vi "总氮质控流程.vi"(6 "队列输入TN":refnum<queue>, 9 "总氮":bool, 10 "总氮量程切换":enum32{"H", "L", "AUTO"}(ring)=enum."AUTO") -> (2 "总氮中断报警":bool, 3 "布尔":bool)   [LabVIEW 2016]
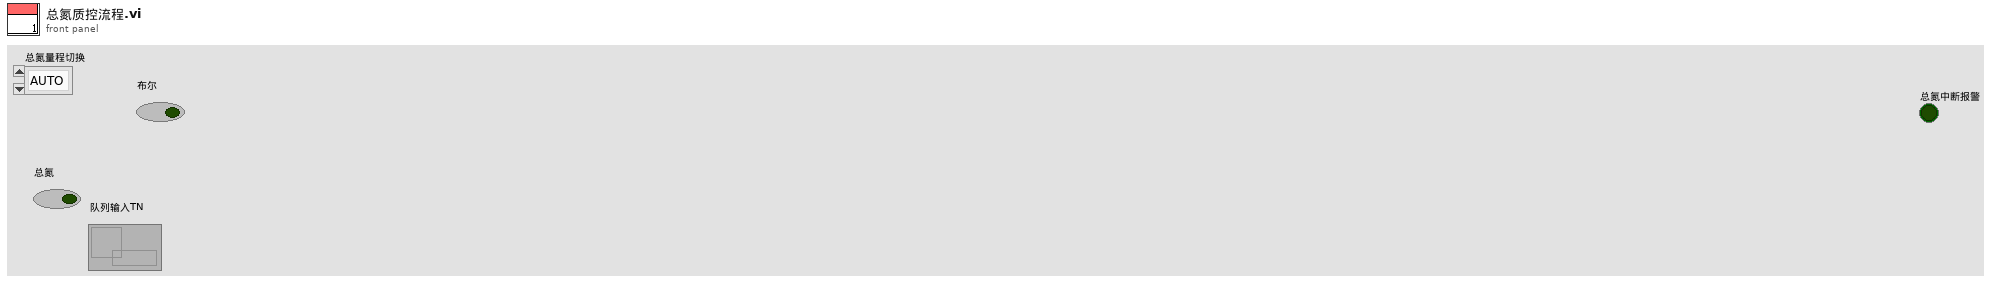
[diagram p1: front panel]
types:
  T1 = enum16{"待机", "启动氨氮水样", "氨氮测量中", "启动氨氮加标", "启动氨氮加标回收", "氨氮加标回收测量中", "启动总氮水样", "总氮测量中", "启动总氮加标", "启动总氮加标回收", "总氮加标回收测量中", "启动总磷水样", "总磷水样测量中", "启动总磷加标", "启动总磷加标回收", "总磷加标回收测量中", "结束"}
  T2 = cluster{"站号":u16, "量程切换":enum32{"H", "L", "AUTO"}, "控制命令":enum16{"启动测量", "标样核查", "零点核查", "跨度核查", "空白测试", "平行样测试", "加标回收", "空白校准", "标样校准", "初始化（清洗）", "停止测试", "仪器重启", "校时", "模式设置", "测量间隔设置"}, "模式设置":enum16{"待机", "连续模式", "周期模式", "定点模式", "受控模式", "手动模式"}, "测量间隔":u16}
  T3 = cluster{"时间标识":timestamp, "设备":string, "日志信息":string}
  T4 = cluster{"系统时间":timestamp, "工作状态":enum16{"空闲", "水样测试", "标样核查", "零点核查", "跨度核查", "空白测试", "平行样测试", "加标回收", "空白校准", "标样校准", "初始化（清洗）"}, "测量模式":enum16{"待机", "连续模式", "周期模式", "定点模式", "受控模式", "手动模式"}, "告警代码":enum16{"无告警", "缺试剂告警", "缺水样告警", "缺蒸馏水告警", "缺标液告警", "仪表漏液告警", "标定异常告警", "超量程告警", "加热异常", "低试剂预警", "超上限告警", "超下限告警", "仪表内部其他异常", "滴定异常告警", "电极异常告警", "量程切换告警", "参数设置告警", "PH电极电位异常", "电导率电极异常", "浊度光度异常", "溶解氧电极异常", "溶解氧光强异常", "温度异常告警", "PH异常告警", "溶解氧异常告警", "电导率异常告警", "浊度异常告警", "叶绿素异常告警", "藻密度异常告警", "蓝绿藻异常告警", "ORP异常告警", "氨氮异常告警", "清洁刷异常告警", "SD卡异常告警", "蓝牙异常告警", "Wifi异常告警", "流程异常告警"}, "故障代码":enum16{"无故障", "电机故障", "温度故障", "通讯故障", "滴定故障"}, "日志代码":u16, "软件版本":u16, "F0":sgl, "F1":sgl, "F2":sgl, "F3":sgl, "T":sgl, "H":sgl, "id":u16, "flowid":u16, "量程":u16, "总磷控温温度1":sgl, "营养盐控温温度2":sgl, "ADC":sgl}
  T5 = enum16{"空闲", "水样测试", "标样核查", "零点核查", "跨度核查", "空白测试", "平行样测试", "加标回收", "空白校准", "标样校准", "初始化（清洗）"}
  T6 = cluster{"因子编码":u32, "单位":u16, "标样参考值":sgl, "水样数据时间":timestamp, "水样实测值":sgl, "水样数据标识":string, "标样数据时间":timestamp, "标样实测值":sgl, "标样数据标识":string, "空白数据时间":timestamp, "空白实测值":sgl, "空白数据标识":string, "零点核查数据时间":timestamp, "零点核查实测值":sgl, "零点核查数据标识":string, "跨度核查数据时间":timestamp, "跨度核查实测值":sgl, "跨度核查数据标识":string, "加标回收数据时间":timestamp, "加标回收实测值":sgl, "加标回收数据标识":string, "平行样数据时间":timestamp, "平行样实测值":sgl, "平行样数据标识":string}
  T7 = cluster{"量程":dbl, "检出限":dbl, "加标前水样浓度":dbl, "加标后水样浓度":dbl, "加标水杯定容体积":dbl, "加标母液浓度":dbl, "加标体积":dbl, "加标回收率":dbl}
  T8 = cluster{"氨氮":u8, "总磷":u8, "总氮":u8, "CODMn":u8, "CODCr":u8}
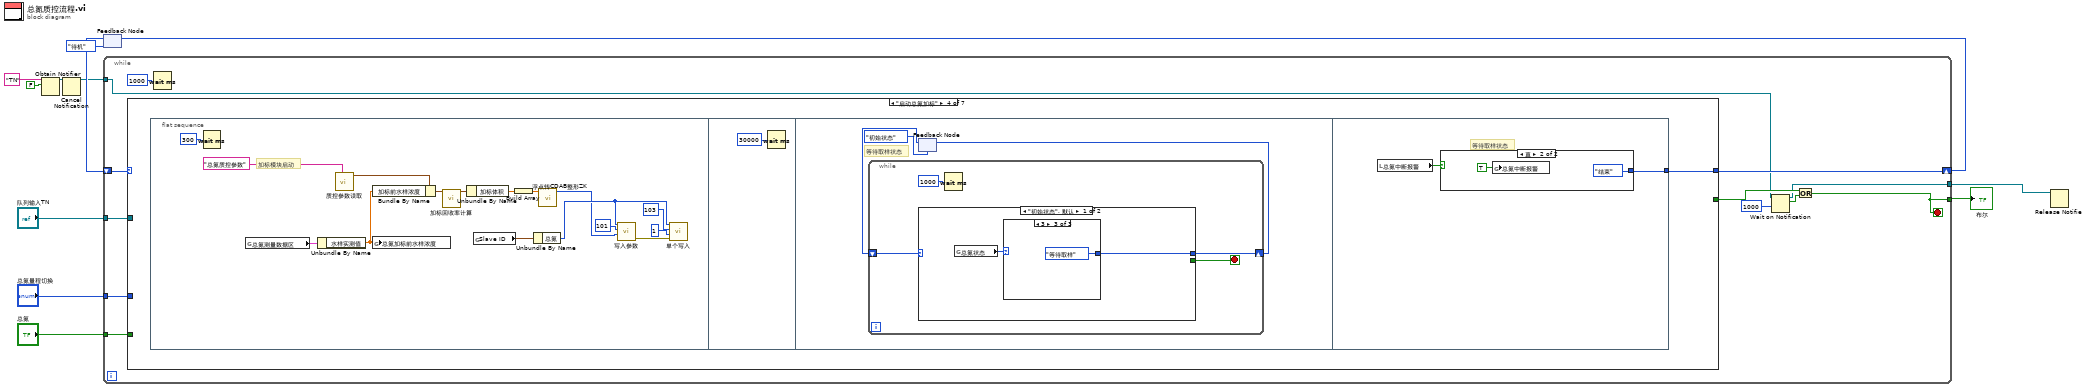
[diagram p0: block diagram]
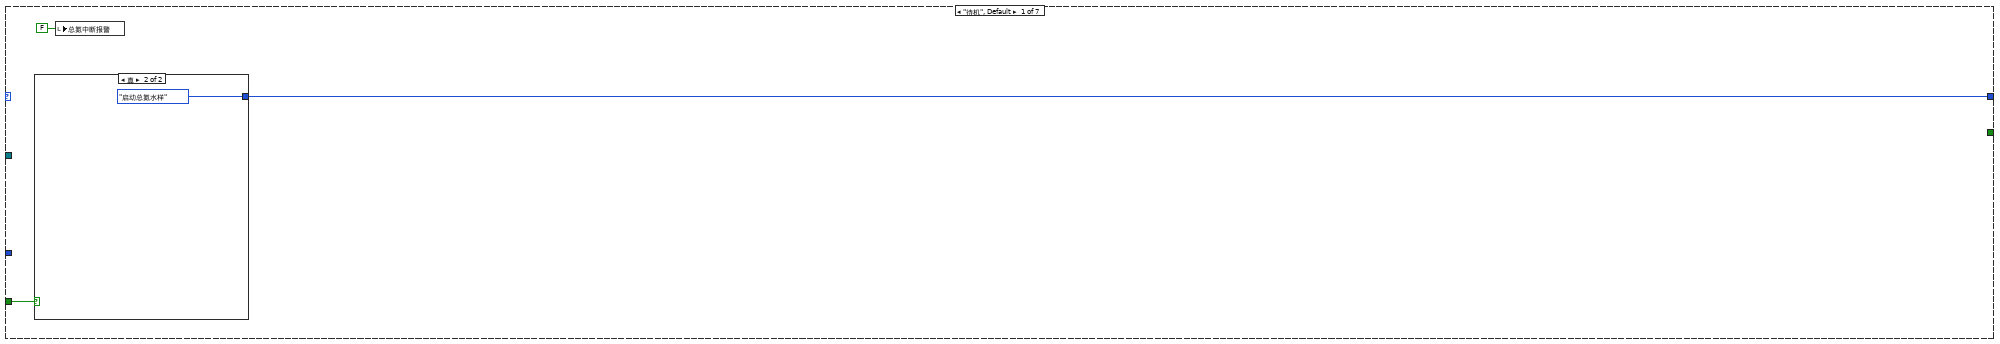
[diagram p2: hidden frame]
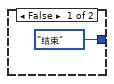
[diagram p3: hidden frame]
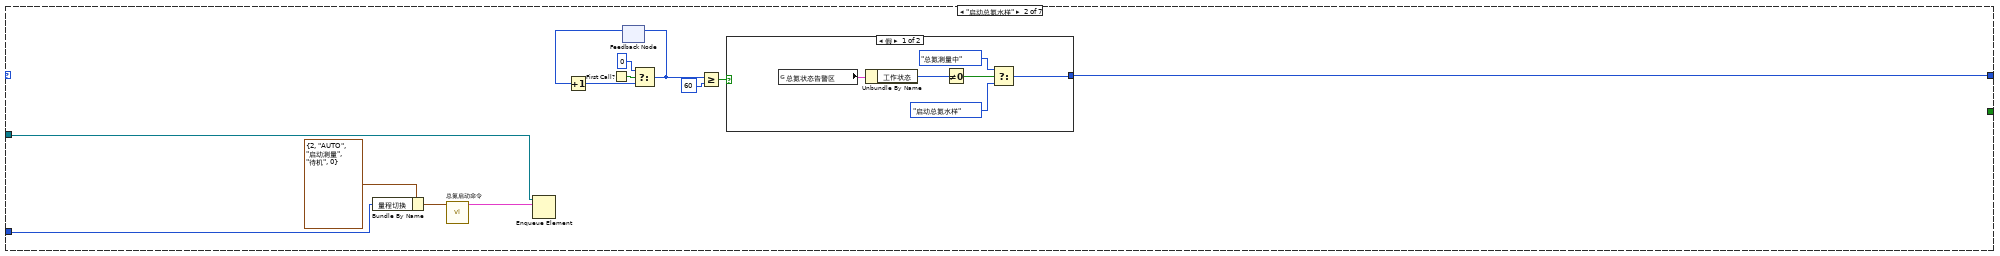
[diagram p4: hidden frame]
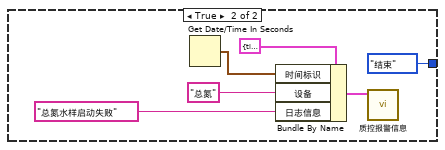
[diagram p5: hidden frame]
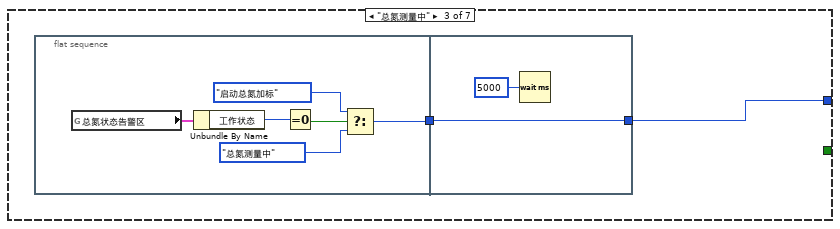
[diagram p6: hidden frame]
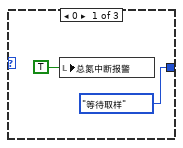
[diagram p7: hidden frame]
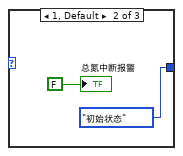
[diagram p8: hidden frame]
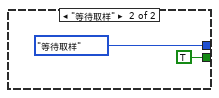
[diagram p9: hidden frame]
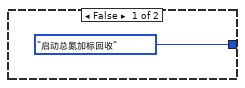
[diagram p10: hidden frame]
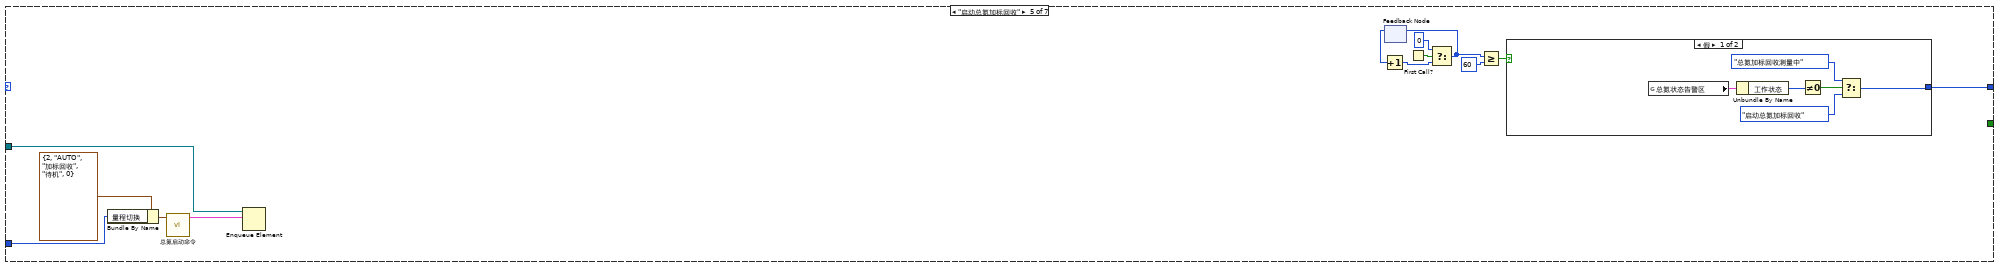
[diagram p11: hidden frame]
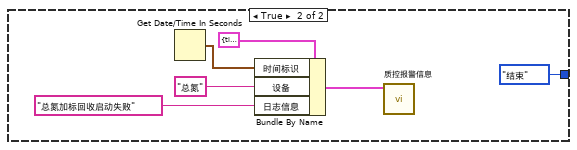
[diagram p12: hidden frame]
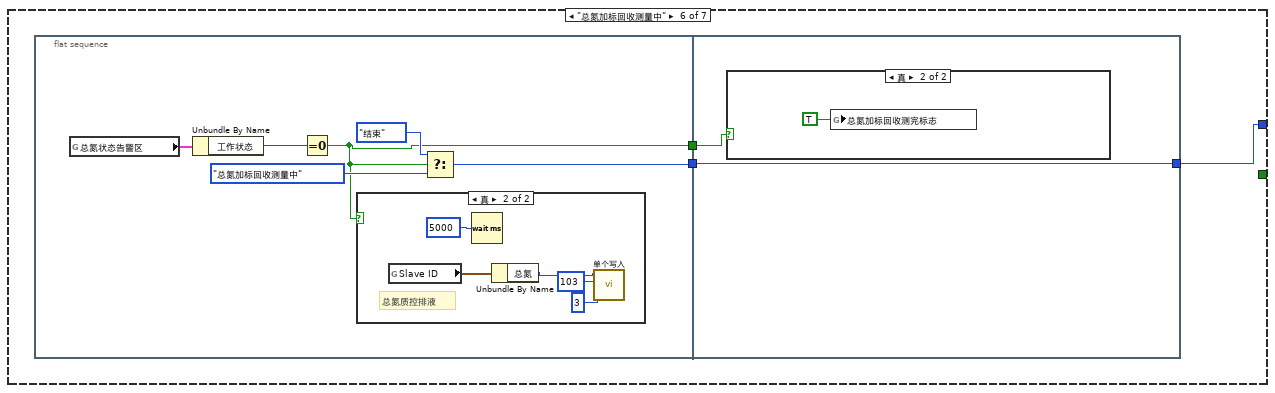
[diagram p13: hidden frame]
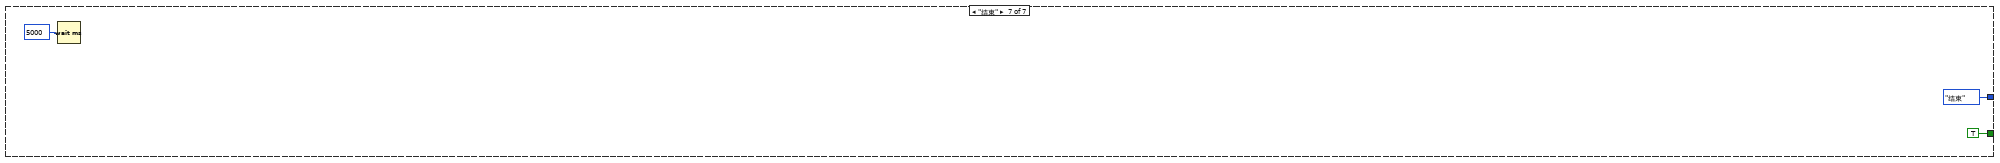
[diagram p16: hidden frame]
diagram:
  n1 = Obtain Notifier(name (unnamed)="TN" ("名称（未命名）"), notification data type=FALSE) -> (notifier out=w3:refnum<notifier>)  [unwired: 2 in, 2 out]
  n2 = Cancel Notification(0:w3) -> (8:w2:refnum<notifier>)  [unwired: 1 in, 2 out]
  n3 = feedback #1(T1."待机") -> (w6:T1)
  n4 = while {
    tunnel: "队列输入TN" -> [w22]
    tunnel: "总氮量程切换" -> [w21]
    tunnel: "总氮" -> [w24]
    tunnel: [w16] -> w11
    shift-right: [w23] -> w9
    shift-left: w6 -> [w20]
    tunnel: w2 -> [w14]
    tunnel: [w15] -> w1
    stop <- w16 stop-if-true
    n5 = case shown="\"启动总氮加标\"" w20 {
      tunnel: [w27 w42 w55 w65 w109 w130 T1."结束"] -> w23
      tunnel: [_ _ _ _ _ _ TRUE] -> w17
      tunnel: w24 -> [w26 _ _ _ _ _ _]
      tunnel: w22 -> [_ w41 _ _ w108 _ _]
      tunnel: w21 -> [_ w40 _ _ w105 _ _]
      frame "待机", Default {
        n6 = case shown="真" w26 {
          tunnel: [T1."结束" T1."启动总氮水样"] -> w27
          frame False {
          }
          frame True {
          }
        }
        n7 = local write "总氮中断报警"(FALSE ("氨氮中断报警")) -> ()
      }
      frame "启动总氮水样" {
        n8 = Bundle By Name(cluster=T2 {"站号"=2, "量程切换"=enum."AUTO", "控制命令"=enum."启动测量", "模式设置"=enum."待机", "测量间隔"=0} ("参数"), "量程切换"=w40) -> (w32:T2)
        n9 = call "总氮启动命令.vi"("参数"=w32) -> ("启动命令"=w30:cluster{"命令":string, "data":variant})  [unwired: 10 in]
        n10 = Enqueue Element(queue=w41, element=w30) -> ()  [unwired: 2 in, 3 out]
        n11 = First Call?() -> (First Call?: T/F=w38:bool)
        n12 = feedback #2() -> (w37:i32)  [unwired: 1 in]
        n13 = Increment(x=w37) -> (x+1=w36:i32)
        n14 = Select(t=0, s=w38, f=w36) -> (s? t:f=w35:i32)
        n15 = feedback-in #2(w35) -> ()
        n16 = Greater Or Equal?(x=w35, y=60) -> (x >= y?=w33:bool)
        n17 = case shown="假" w33 {
          tunnel: [w47 T1."结束"] -> w42
          frame False {
            n18 = global read "与总氮交互全局.vi" "总氮状态告警区"() -> (w44:T4)
            n19 = Unbundle By Name(w44) -> ("工作状态"=w43:T5)
            n20 = Not Equal To 0?(x=w43) -> (x != 0?=w48:bool)
            n21 = Select(t=T1."总氮测量中", s=w48, f=T1."启动总氮水样") -> (s? t:f=w47:T1)
          }
          frame True {
            n22 = Get Date/Time In Seconds() -> (seconds since 1Jan1904=w54:timestamp)
            n23 = Bundle By Name(cluster=T3 {"时间标识"=timestamp(0 s since 1904-01-01), "设备"="", "日志信息"=""} ("data in"), "时间标识"=w54, "设备"="总氮", "日志信息"="总氮水样启动失败") -> (w49:T3)
            n24 = call "质控报警信息.vi"("data in"=w49) -> ()  [unwired: 11 in]
          }
        }
      }
      frame "总氮测量中" {
        n25 = flat-sequence {
          tunnel: [w57] -> w56
          tunnel: w56 -> [w63]
          tunnel: [w63] -> w55
          frame #0 {
            n26 = global read "与总氮交互全局.vi" "总氮状态告警区"() -> (w62:T4)
            n27 = Unbundle By Name(w62) -> ("工作状态"=w61:T5)
            n28 = Equal To 0?(x=w61) -> (x = 0?=w60:bool)
            n29 = Select(t=T1."启动总氮加标", s=w60, f=T1."总氮测量中") -> (s? t:f=w57:T1)
          }
          frame #1 {
            n30 = Wait (ms)(milliseconds to wait=u32 5000 ("等待时间（毫秒）")) -> ()  [unwired: 1 out]
          }
        }
      }
      frame "启动总氮加标" {
        n31 = flat-sequence {
          tunnel: [w100] -> w65
          frame #0 {
            # "加标模块启动"
            n32 = Wait (ms)(milliseconds to wait=u32 300 ("等待时间（毫秒）")) -> ()  [unwired: 1 out]
            n33 = global read "与总氮交互全局.vi" "总氮测量数据区"() -> (w74:T6)
            n34 = Unbundle By Name(w74) -> ("水样实测值"=w76:sgl)
            n35 = call "质控参数读取.vi"("section"="总氮质控参数") -> ("参数"=w79:T7)  [unwired: 9 in, 1 out]
            n36 = Bundle By Name(cluster=w79, "加标前水样浓度"=w76) -> (w80:T7)
            n37 = global write "水样浓度全局.vi" "总氮加标前水样浓度"(w76) -> ()
            n38 = call "加标回收率计算.vi"("参数"=w80) -> ("参数 out"=w78:T7)  [unwired: 9 in, 1 out]
            n39 = Unbundle By Name(w78) -> ("加标体积"=w77:dbl)
            n40 = global read "断电保存全局.vi" "Slave ID"() -> (w72:T8)
            n41 = Build Array(w77) -> (w73:dbl[])
            n42 = Unbundle By Name(w72) -> ("总氮"=w67:u8)
            n43 = call "浮点转CDAB整形ZK.vi"("浮点数"=w73) -> ("CDAB整形输出"=w66:u16[])  [unwired: 10 in]
            n44 = call "写入参数.vi"("values"=w66, "starting address"=u16 101, "Slave ID"=w67) -> ("error out"=w71:errorcluster)  [unwired: 8 in]
            n45 = call "单个写入.vi"("Error in"=w71, "value"=u16 1, "address"=u16 103, "Slave ID"=w67) -> ()  [unwired: 7 in, 1 out]
          }
          frame #1 {
            n46 = Wait (ms)(milliseconds to wait=u32 30000 ("等待时间（毫秒）")) -> ()  [unwired: 1 out]
          }
          frame #2 {
            # "等待取样状态"
            n47 = feedback #3(enum16{"初始状态", "等待取样"}."初始状态") -> (w84:enum16{"初始状态", "等待取样"})
            n48 = while {
              shift-right: [w88] -> w85
              shift-left: w84 -> [w89]
              stop <- w87 stop-if-true
              n49 = case shown="\"初始状态\", 默认" w89 {
                tunnel: [w91 enum16{"初始状态", "等待取样"}."等待取样"] -> w88
                tunnel: [_ TRUE] -> w87
                frame "初始状态", Default {
                  n50 = global read "加标回收状态全局变量.vi" "总氮状态"() -> (w90:u16)
                  n51 = case shown="3" w90 {
                    tunnel: [enum16{"初始状态", "等待取样"}."等待取样" enum16{"初始状态", "等待取样"}."初始状态" enum16{"初始状态", "等待取样"}."等待取样"] -> w91
                    frame 0 {
                      n52 = local write "总氮中断报警"(TRUE ("氨氮中断报警")) -> ()
                    }
                    frame 1, Default {
                      "总氮中断报警" <- FALSE ("总氮中断报警")
                    }
                    frame 3 {
                    }
                  }
                }
                frame "等待取样" {
                }
              }
              n53 = Wait (ms)(milliseconds to wait=u32 1000 ("等待时间（毫秒）")) -> ()  [unwired: 1 out]
            }
            n54 = feedback-in #3(w85) -> ()
          }
          frame #3 {
            # "等待取样状态"
            n55 = local read "总氮中断报警"() -> (w99:bool)
            n56 = case shown="真" w99 {
              tunnel: [T1."启动总氮加标回收" T1."结束"] -> w100
              frame False {
              }
              frame True {
                n57 = global write "质控中断报警全局.vi" "总氮中断报警"(TRUE ("总氮中断报警")) -> ()
              }
            }
          }
        }
      }
      frame "启动总氮加标回收" {
        n58 = Bundle By Name(cluster=T2 {"站号"=2, "量程切换"=enum."AUTO", "控制命令"=enum."加标回收", "模式设置"=enum."待机", "测量间隔"=0} ("参数"), "量程切换"=w105) -> (w107:T2)
        n59 = call "总氮启动命令.vi"("参数"=w107) -> ("启动命令"=w104:cluster{"命令":string, "data":variant})  [unwired: 10 in]
        n60 = Enqueue Element(queue=w108, element=w104) -> ()  [unwired: 2 in, 3 out]
        n61 = feedback #4() -> (w114:i32)  [unwired: 1 in]
        n62 = Increment(x=w114) -> (x+1=w113:i32)
        n63 = First Call?() -> (First Call?: T/F=w115:bool)
        n64 = Select(t=0, s=w115, f=w113) -> (s? t:f=w112:i32)
        n65 = feedback-in #4(w112) -> ()
        n66 = Greater Or Equal?(x=w112, y=60) -> (x >= y?=w110:bool)
        n67 = case shown="假" w110 {
          tunnel: [w120 T1."结束"] -> w109
          frame False {
            n68 = global read "与总氮交互全局.vi" "总氮状态告警区"() -> (w117:T4)
            n69 = Unbundle By Name(w117) -> ("工作状态"=w122:T5)
            n70 = Not Equal To 0?(x=w122) -> (x != 0?=w121:bool)
            n71 = Select(t=T1."总氮加标回收测量中", s=w121, f=T1."启动总氮加标回收") -> (s? t:f=w120:T1)
          }
          frame True {
            n72 = Get Date/Time In Seconds() -> (seconds since 1Jan1904=w128:timestamp)
            n73 = Bundle By Name(cluster=T3 {"时间标识"=timestamp(0 s since 1904-01-01), "设备"="", "日志信息"=""} ("data in"), "时间标识"=w128, "设备"="总氮", "日志信息"="总氮加标回收启动失败") -> (w123:T3)
            n74 = call "质控报警信息.vi"("data in"=w123) -> ()  [unwired: 11 in]
          }
        }
      }
      frame "总氮加标回收测量中" {
        n75 = flat-sequence {
          tunnel: [w136] -> w131
          tunnel: [w132] -> w129
          tunnel: [w144] -> w130
          tunnel: w131 -> [w144]
          tunnel: w129 -> [w143]
          frame #0 {
            n76 = global read "与总氮交互全局.vi" "总氮状态告警区"() -> (w133:T4)
            n77 = Unbundle By Name(w133) -> ("工作状态"=w137:T5)
            n78 = Equal To 0?(x=w137) -> (x = 0?=w132:bool)
            n79 = case shown="真" w132 {
              frame False {
              }
              frame True {
                # "总氮质控排液"
                n80 = global read "断电保存全局.vi" "Slave ID"() -> (w141:T8)
                n81 = Wait (ms)(milliseconds to wait=u32 5000 ("等待时间（毫秒）")) -> ()  [unwired: 1 out]
                n82 = Unbundle By Name(w141) -> ("总氮"=w138:u8)
                n83 = call "单个写入.vi"("value"=u16 3, "address"=u16 103, "Slave ID"=w138) -> ()  [unwired: 8 in, 1 out]
              }
            }
            n84 = Select(t=T1."结束", s=w132, f=T1."总氮加标回收测量中") -> (s? t:f=w136:T1)
          }
          frame #1 {
            n85 = case shown="真" w143 {
              frame False {
              }
              frame True {
                n86 = global write "质控测完标志全局 1.vi" "总氮加标回收测完标志"(TRUE) -> ()
              }
            }
          }
        }
      }
      frame "结束" {
        n87 = Wait (ms)(milliseconds to wait=u32 5000 ("等待时间（毫秒）")) -> ()  [unwired: 1 out]
      }
    }
    n88 = Wait (ms)(milliseconds to wait=u32 1000 ("等待时间（毫秒）")) -> ()  [unwired: 1 out]
    n89 = Wait on Notification(notifier=w14, timeout in ms (-1)=1000 ("超时毫秒(-1)")) -> (notifier out=w15:refnum<notifier>, notification=w18:bool)  [unwired: 2 in, 2 out]
    n90 = Or(x=w17, y=w18) -> (x .or. y?=w16:bool)
  }
  "布尔" <- w11
  n91 = feedback-in #1(w9) -> ()
  n92 = Release Notifier(notifier=w1) -> ()  [unwired: 2 in, 3 out]
